vi "LV SciSDK RATEMETER.vi"(7 "Ratemeter Handle In":T3, 9 "Board Handle In":T1, 11 "error in (no error)":errorcluster) -> (4 "NI Error Code":i32, 6 "Ratemeter Buffer Out":T2, 8 "Ratemeter Handle Out":T3, 10 "Board Handle Out":T1, 15 "error out":errorcluster)   [LabVIEW 2021, in "SciSDK_Labview.lvlib"]
uses:
  SciSDK_Labview.lvlib
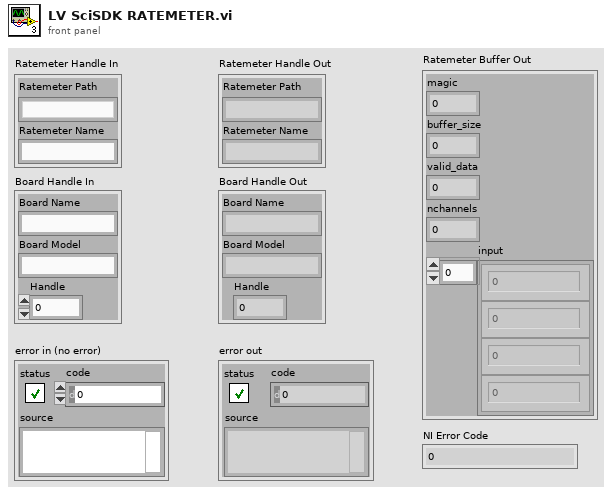
[diagram p1: front panel]
types:
  T1 = cluster{"Board Name":string, "Board Model":string, "Handle":u64}
  T2 = cluster{"magic":u32, "buffer_size":u32, "valid_data":u32, "nchannels":u32, "input":dbl[]}
  T3 = cluster{"Ratemeter Path":string, "Ratemeter Name":string}
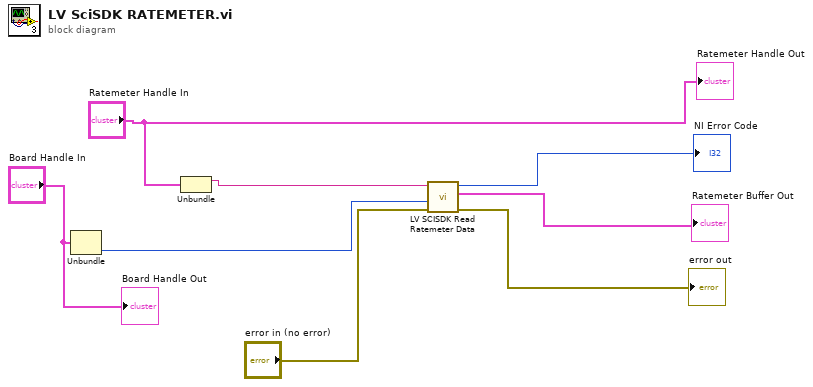
[diagram p0: block diagram]
diagram:
  n1 = Unbundle("Board Handle In") -> ("Handle"=w2:u64)  [unwired: 2 out]
  n2 = Unbundle("Ratemeter Handle In") -> ("Ratemeter Path"=w3:string)  [unwired: 1 out]
  n3 = call "LV SCISDK Read Ratemeter Data.vi"("Path"=w3, "handle"=w2, "error in (no error)"="error in (no error)") -> ("function return"=→"NI Error Code":i32, "buffer out"=→"Ratemeter Buffer Out":T2, "error out"=→"error out":errorcluster)  [unwired: 4 in, 1 out]
  "Ratemeter Handle Out" <- "Ratemeter Handle In"
  "Board Handle Out" <- "Board Handle In"
